vi "Get Request Type.vi"(8 "error in (no error)":errorcluster, 11 "GetProfileParameter in":refnum<class "GetProfileParameter.lvclass">) -> (0 "error out":errorcluster, 2 "Request Type":string, 3 "GetProfileParameter out":refnum<class "GetProfileParameter.lvclass">)   [LabVIEW 2020, in "obs-websocket.lvlib" / "GetProfileParameter.lvclass"]
uses:
  GetProfileParameter.lvclass
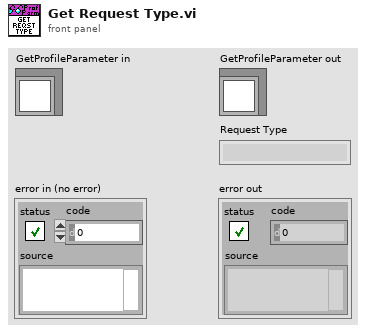
[diagram p1: front panel]
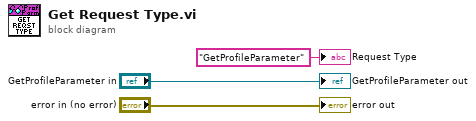
[diagram p0: block diagram]
diagram:
  "error out" <- "error in (no error)"
  "GetProfileParameter out" <- "GetProfileParameter in"
  "Request Type" <- "GetProfileParameter" ("Request Type")
